vi "Hardware Scan.vi"(8 "error in (no error)":errorcluster, 11 "TestStand Controller in":refnum<class "Controller API.lvclass">) -> (0 "error out":errorcluster, 3 "TestStand Controller out":refnum<class "Controller API.lvclass">)   [LabVIEW 2016, in "Controller API.lvlib" / "Controller API.lvclass"]
uses:
  <userlib>/Measurement Utility API/Controller API.lvclass
  C:/Program Files (x86)/National Instruments/LabVIEW 2016/user.lib/Common Components/Controller/Controller.lvclass
  <userlib>/Common Components/Controller/Controller.lvclass/Controller.ctl
  <userlib>/Common Components/Controller/Accessors/Read Root Path.vi
  <userlib>/Common Components/Controller/Controller.lvclass
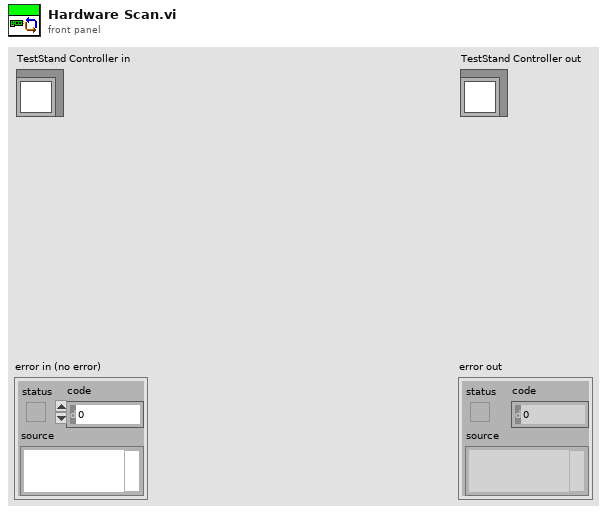
[diagram p1: front panel]
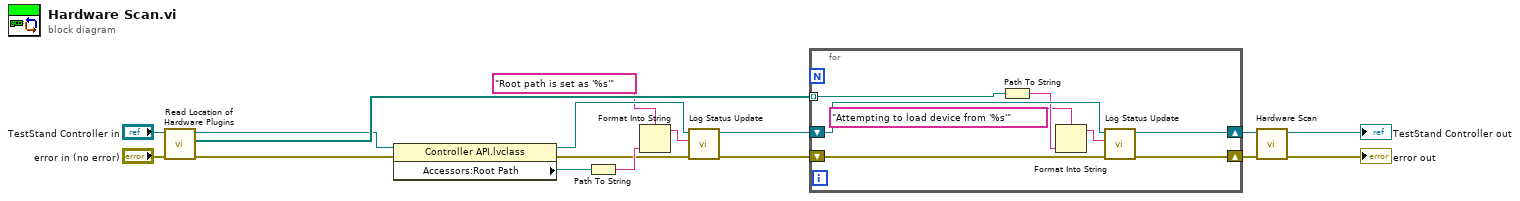
[diagram p0: block diagram]
diagram:
  n1 = call <userlib>:"Read Location of Hardware Plugins.vi"("error in (no error)"="error in (no error)", "Controller in"="TestStand Controller in") -> ("error out"=w8:errorcluster, "Array of Hardware Paths"=w16:path[], "Controller out"=w15:refnum<class "Controller API.lvclass">)  [unwired: 7 in]
  n2 = property class="Controller API.lvclass"(reference=w15, error in=w8) -> (reference out=w13:refnum<class "Controller API.lvclass">, error out=w7:errorcluster, "Accessors:Root Path"=w12:path)
  n3 = Path To String(path=w12) -> (string=w10:string)
  n4 = Format Into String(format string="Root path is set as '%s'", w10) -> (resulting string=w9:string)  [unwired: 2 in, 1 out]
  n5 = call-dynamic "Log Status Update.vi"("error in (no error)"=w7, "String"=w9, "TestStand Controller in"=w13) -> ("error out"=w6:errorcluster, "TestStand Controller out"=w14:refnum<class "Controller API.lvclass">)  [unwired: 7 in]
  n6 = for {
    tunnel: w16 -> [w25] mode=indexing
    shift-right: [w23] -> w4
    shift-left: w14 -> [w24]
    shift-right: [w18] -> w1
    shift-left: w6 -> [w19]
    n7 = Path To String(path=w25) -> (string=w21:string)
    n8 = Format Into String(format string="Attempting to load device from '%s'", w21) -> (resulting string=w22:string)  [unwired: 2 in, 1 out]
    n9 = call-dynamic "Log Status Update.vi"("error in (no error)"=w19, "String"=w22, "TestStand Controller in"=w24) -> ("error out"=w18:errorcluster, "TestStand Controller out"=w23:refnum<class "Controller API.lvclass">)  [unwired: 7 in]
  }
  n10 = call-parent "Hardware Scan.vi"("error in (no error)"=w1, "Controller in"=w4) -> ("error out"=→"error out":errorcluster, "Controller out"=→"TestStand Controller out":refnum<class "Controller API.lvclass">)  [unwired: 8 in]
